vi "setEOTParameters.vi"(0 "connection ID":refnum<k5>, 5 "axis [0|1|2]":u8, 7 "minAvgStepSize_nm":i32, 9 "numOfAvgedSteps":i32, 11 "error":errorcluster) -> (4 "connection ID out":refnum<k5>, 6 "axis out":u8, 15 "error out":errorcluster)   [LabVIEW 2016, in "AMC_VIs.lvlib"]
doc: "This function sets the parameters for the EOT-detection\nInputs:\n -- connection string (from connect_TCP.vi)\n -- axis [0|1|2]\n -- minAvgStepSize_nm: minimal averaged step-size, that is still not interpreted as eot\n-- numOfAvgedSteps: number of steps, that are averaged to calculate the minAvgStepSize\n\nOutputs:\n -- error\n -- connection ID out\n -- axis out"
uses:
  AMC_VIs.lvlib
panel:
  out "JSON-response":string="{\"jsonrpc\":\"2.0\",\"method\":\"\",\"params\":[5,1.245,true,\"name\"],\"id\":\"1\"}"
  out "JSON request":string
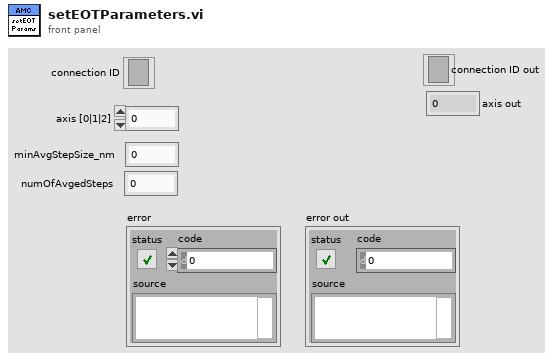
[diagram p1: front panel]
types:
  T1 = cluster{"jsonrpc":string, "method":string, "params":i32[], "id":string, "api":string}
  T2 = cluster{"jsonrpc":string, "result":i32[], "id":string}
  T3 = enum16{"Standard", "Buffered", "CRLF", "Immediate"}
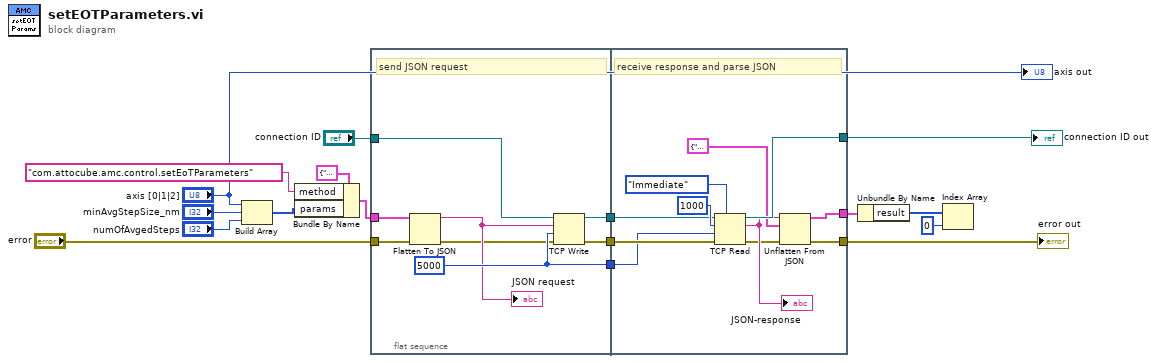
[diagram p0: block diagram]
diagram:
  n1 = Build Array("axis [0|1|2]", "minAvgStepSize_nm", "numOfAvgedSteps") -> (w9:i32[])
  n2 = Bundle By Name(cluster=T1 {"jsonrpc"="2.0", "method"="com.attocube.amc.res.setRESReadOutFreq", "params"=[0, 2712], "id"="1", "api"="2"} ("InputParams 2"), "method"="com.attocube.amc.control.setEoTParameters", "params"=w9) -> (w8:T1)
  n3 = flat-sequence {
    tunnel: "connection ID" -> [w25]
    tunnel: [w23] -> w17
    tunnel: [w24] -> w16
    tunnel: "error" -> [w19]
    tunnel: [w22] -> w15
    tunnel: w8 -> [w21]
    tunnel: [w32] -> w1
    tunnel: w17 -> [w34]
    tunnel: w16 -> [w33]
    tunnel: [w28] -> w2
    tunnel: w15 -> [w31]
    tunnel: [w27] -> w7
    frame #0 {
      w22 = 5000 ("timeout ms (25000)")
      # "send JSON request"
      n4 = Flatten To JSON(anything=w21, error in (no error)=w19) -> (JSON string=w20:string, 11:w18:errorcluster)  [unwired: 1 in]
      "JSON request" <- w20
      n5 = TCP Write(connection ID=w25, data in=w20, error in (no error)=w18, 9:w22) -> (connection ID out=w23:refnum<k5>, error out=w24:errorcluster)  [unwired: 1 out]
    }
    frame #1 {
      # "receive response and parse JSON"
      n6 = TCP Read(connection ID=w34, bytes to read=1000, error in (no error)=w33, 7:T3."Immediate" ("mode (standard)"), 9:w31) -> (connection ID out=w32:refnum<k5>, data out=w30:string, error out=w29:errorcluster)
      "JSON-response" <- w30
      n7 = Unflatten From JSON(JSON string=w30, type and defaults=T2 {"jsonrpc"="2.0", "result"=[0, 2712], "id"="1"} ("InputParams 2"), error in (no error)=w29) -> (value=w27:T2, error out=w28:errorcluster)  [unwired: 4 in]
    }
  }
  n8 = Unbundle By Name(w7) -> ("result"=w5:i32[])
  n9 = Index Array(array=w5, index=0) -> ()  [unwired: 1 out]
  "error out" <- w2
  "connection ID out" <- w1
  "axis out" <- "axis [0|1|2]"
